vi "New Database path.vi"(10 "Database Name":string) -> (2 "Database path":path)   [LabVIEW 2019]
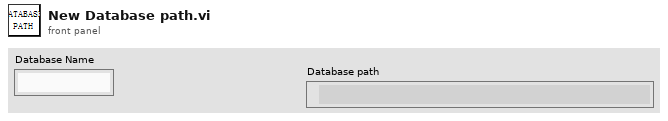
[diagram p1: front panel]
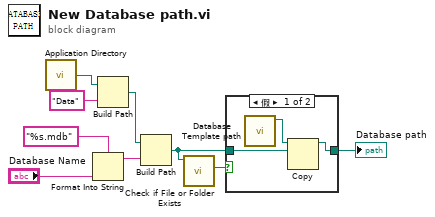
[diagram p0: block diagram]
diagram:
  n1 = call <vilib>:"Application Directory.vi"() -> ("Application Directory"=w7:path)
  n2 = Format Into String(format string="%s.mdb" ("格式字符串"), "Database Name") -> (resulting string=w4:string)  [unwired: 2 in, 1 out]
  n3 = Build Path(base path=w7, name or relative path="Data" ("名称或相对路径")) -> (appended path=w5:path)
  n4 = Build Path(base path=w5, name or relative path=w4) -> (appended path=w2:path)
  n5 = call <vilib>:"Check if File or Folder Exists.vi"("path"=w2) -> ("file or folder exists?"=w1:bool)  [unwired: 8 in, 2 out]
  n6 = case shown="假" w1 {
    tunnel: [w11 w13] -> w3
    tunnel: w2 -> [w10 w13]
    frame False {
      n7 = call "Database Template path.vi"() -> ("Access path"=w12:path)  [unwired: 11 in]
      n8 = Copy(10:w10, 11:w12) -> (3:w11:path)  [unwired: 3 in, 2 out]
    }
    frame True {
    }
  }
  "Database path" <- w3
